vi "Wrap Value.vi"(9 "Min":sgl, 10 "Max":sgl, 11 "Value":sgl) -> (3 "Wrapped Value":sgl)   [LabVIEW 2021, in "Math.lvlib"]
uses:
  Math.lvlib
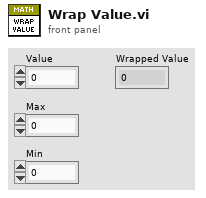
[diagram p1: front panel]
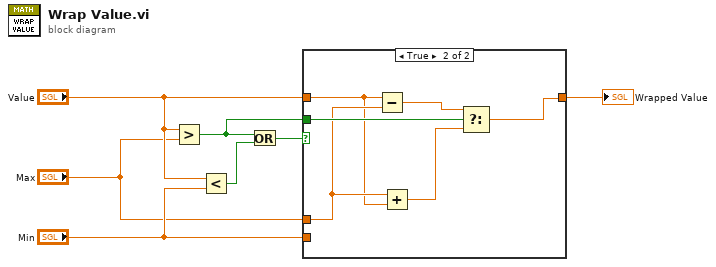
[diagram p0: block diagram]
diagram:
  n1 = Greater?(x="Value", y="Max") -> (0:w1:bool)
  n2 = Less?(x="Value", y="Min") -> (x < y?=w7:bool)
  n3 = Or(x=w1, y=w7) -> (x .or. y?=w6:bool)
  n4 = case shown="True" w6 {
    tunnel: "Value" -> [w8 w10]
    tunnel: [w8 w12] -> w4
    tunnel: "Min" -> [_ _]
    tunnel: "Max" -> [_ w11]
    tunnel: w1 -> [_ w14]
    frame False {
    }
    frame True {
      n5 = Subtract(x=w10, y=w11) -> (x-y=w13:sgl)
      n6 = Add(x=w11, y=w10) -> (x+y=w9:sgl)
      n7 = Select(t=w13, s=w14, f=w9) -> (s? t:f=w12:sgl)
    }
  }
  "Wrapped Value" <- w4
